vi "Add New BD Element.vi"(8 "error in (no error)":errorcluster, 11 "Block Diagram in":T1) -> (0 "error out":errorcluster, 3 "Block Diagram out":T1)   [LabVIEW 2025]
uses:
  Controls/bd.ctl
  Classes/Node/Node.lvclass
  Controls/wire.ctl
  Controls/Terminal.ctl
  <vilib>/Utility/error.llb/DialogType.ctl
  Classes/Node/Node.lvclass/Node.ctl
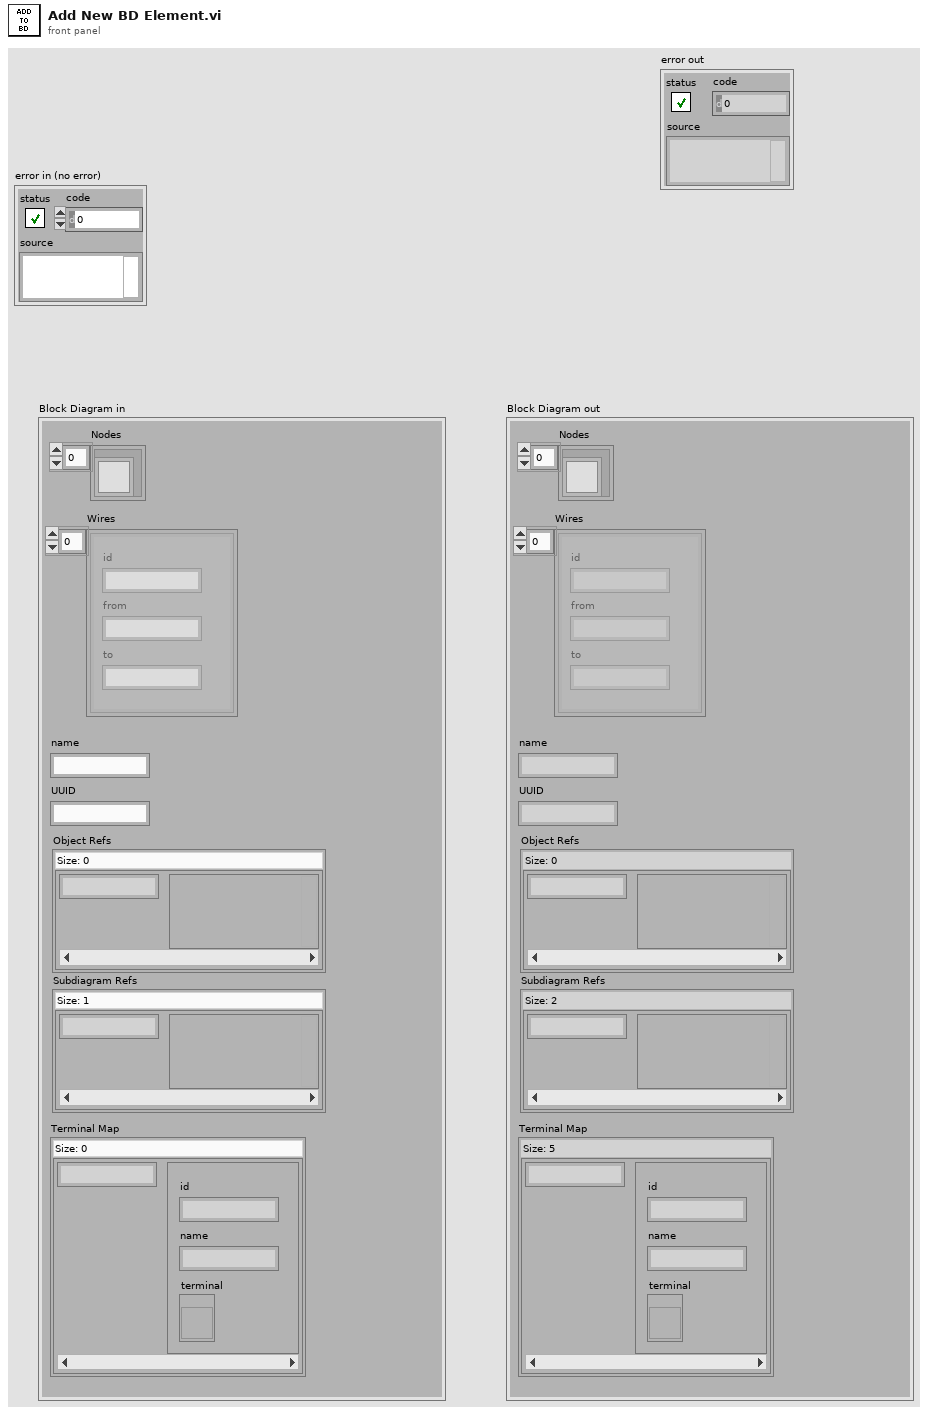
[diagram p1: front panel]
types:
  T1 = typedef "bd.ctl" = cluster{"Nodes":refnum<class "Node.lvclass">[], "Wires":T2[], "name":string, "UUID":string, "Object Refs":map{string, variant}, "Subdiagram Refs":map{string, variant}, "Terminal Map":map{string, T3}}
  T2 = typedef "wire.ctl" = cluster{"id":string, "from":string, "to":string}
  T3 = typedef "Terminal.ctl" = cluster{"id":string, "name":string, "terminal":refnum<vi>}
  T4 = typedef "DialogType.ctl" = u16
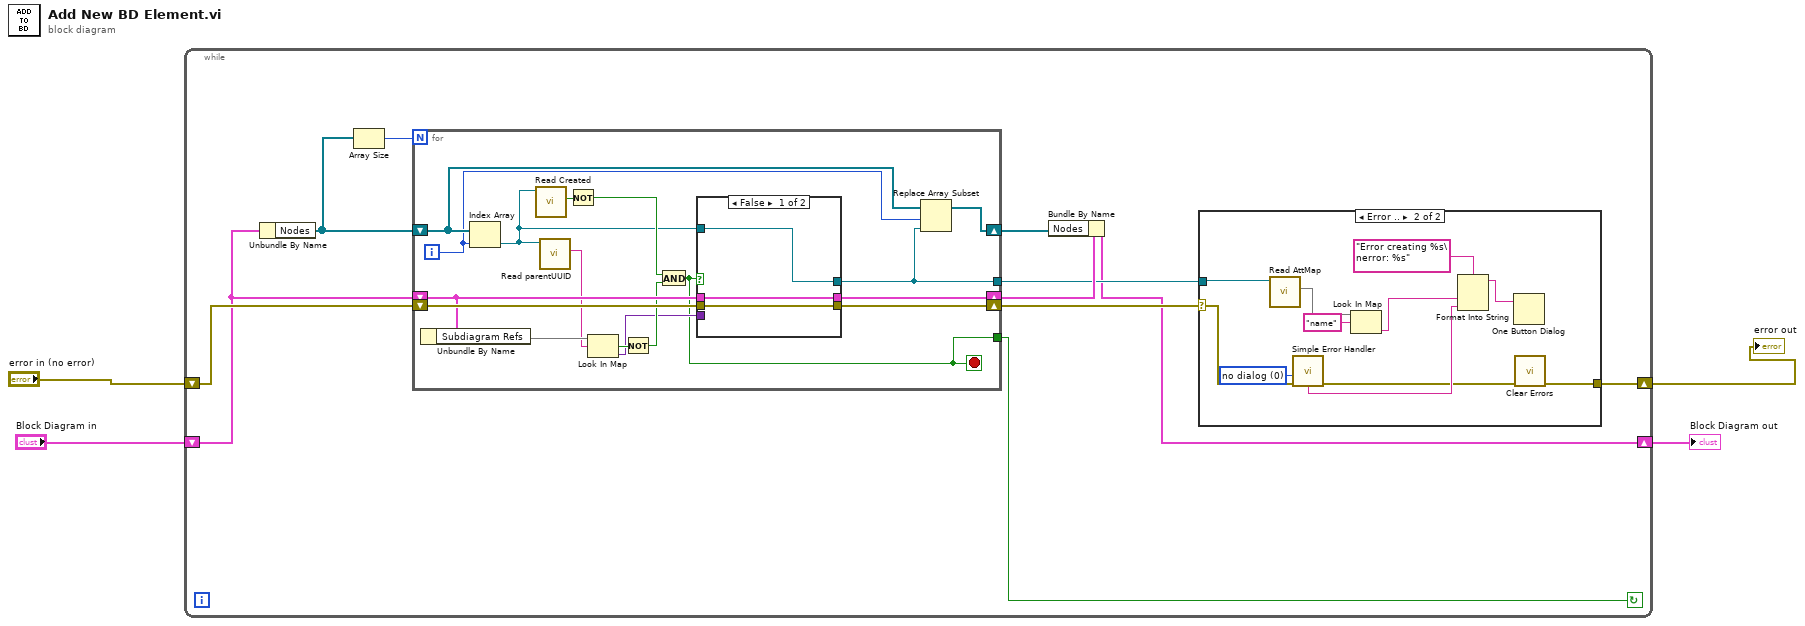
[diagram p0: block diagram]
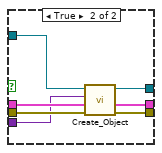
[diagram p2: hidden frame]
diagram:
  n1 = while {
    shift-right: [w7] -> w4
    shift-left: "Block Diagram in" -> [w10]
    shift-right: [w11] -> w1
    shift-left: "error in (no error)" -> [w14]
    stop <- w5 continue-if-true
    n2 = Unbundle By Name(w10) -> ("Nodes"=w8:refnum<class "Node.lvclass">[])
    n3 = Array Size(array=w8) -> (size(s)=w9:i32)
    n4 = for {
      N: w9 -> [_]
      tunnel: [w19] -> w12
      shift-right: [w32] -> w15
      shift-left: w10 -> [w29]
      shift-right: [w30] -> w13
      shift-left: w14 -> [w31]
      shift-right: [w18] -> w6
      shift-left: w8 -> [w21]
      tunnel: [w16] -> w5
      i -> [w20]
      stop <- w16 stop-if-true
      n5 = Unbundle By Name(w29) -> ("Subdiagram Refs"=w28:map{string, variant})
      n6 = Index Array(array=w21, index=w20) -> (element=w22:refnum<class "Node.lvclass">)
      n7 = call-dynamic "Read Created.vi"("Node in"=w22) -> ("Created"=w25:bool)  [unwired: 8 in, 2 out]
      n8 = call-dynamic "Read parentUUID.vi"("Node in"=w22) -> ("parentUUID"=w27:string)  [unwired: 8 in, 2 out]
      n9 = Not(x=w25) -> (.not. x?=w23:bool)
      n10 = Look In Map(map=w28, key=w27) -> (key not found?=w26:bool, value=w17:variant)  [unwired: 1 in]
      n11 = Not(x=w26) -> (.not. x?=w24:bool)
      n12 = And(x=w23, y=w24) -> (x .and. y?=w16:bool)
      n13 = case shown="False" w16 {
        tunnel: [w34 w42] -> w32
        tunnel: w31 -> [w35 w41]
        tunnel: [w35 w40] -> w30
        tunnel: [w33 w39] -> w19
        tunnel: w29 -> [w34 w38]
        tunnel: w22 -> [w33 w37]
        tunnel: w17 -> [_ w36]
        frame False {
        }
        frame True {
          n14 = call-dynamic "Create_Object.vi"("error in (no error)"=w41, "Block Diagram in"=w38, "owner refnum"=w36, "Node in"=w37) -> ("error out"=w40:errorcluster, "Block Diagram Out"=w42:T1, "Node out"=w39:refnum<class "Node.lvclass">)  [unwired: 5 in]
        }
      }
      n15 = Replace Array Subset(array=w21, new element=w19, index=w20) -> (w18:refnum<class "Node.lvclass">[])
    }
    n16 = Bundle By Name(cluster=w15, "Nodes"=w6) -> (w7:T1)
    n17 = case shown="Error .." w13 {
      selector: w13 -> [w43 w48]
      tunnel: w12 -> [_ w53]
      tunnel: [w43 w44] -> w11
      frame No Error {
      }
      frame Error {
        w47 = T4 0 items=["no dialog", "OK message", "continue or stop message", "OK message + warnings", "continue/stop + warnings"] ("type of dialog (OK msg:1)")
        n18 = call "Read AttMap.vi"("Node in"=w53) -> ("AttMap"=w52:map{string, string})  [unwired: 8 in, 2 out]
        n19 = call <vilib>:"Simple Error Handler.vi"("type of dialog (OK msg:1)"=w47, "error in (no error)"=w48) -> ("error out"=w45:errorcluster, "message"=w46:string)  [unwired: 3 in, 3 out]
        n20 = Look In Map(map=w52, key="name") -> (value=w50:string)  [unwired: 1 in, 1 out]
        n21 = Format Into String(format string="Error creating %s\nerror: %s", w50, w46) -> (resulting string=w49:string)  [unwired: 2 in, 1 out]
        n22 = One Button Dialog(message=w49) -> ()  [unwired: 1 in, 1 out]
        n23 = call <vilib>:"Clear Errors.vi"("error in (no error)"=w45) -> ("error out"=w44:errorcluster)  [unwired: 5 in, 1 out]
      }
    }
  }
  "Block Diagram out" <- w4
  "error out" <- w1
